vi "AQI SERIAL VISA.vi"() -> ()   [LabVIEW 2023]
uses:
  <vilib>/Instr/_visa.llb/VISA Configure Serial Port (Instr).vi
panel:
  out "MQ7 SENSOR":i32(graph)
  in  "VISA resource name":refnum<visa-resource-name>
  out "read buffer":string
  out "AIR QUALITY SENSOR":dbl(knob) scale=0.0..400.0
  out "GAS METER":dbl(knob) scale=0.0..400.0
  out "CO METER":dbl(slide) scale=0.0..400.0
  out "MQ135 SENSOR":i32(graph)
  out "MQ4 SENSOR":i32(graph)
  in  "STOP":bool
  # "AmanKapil_21001017005"
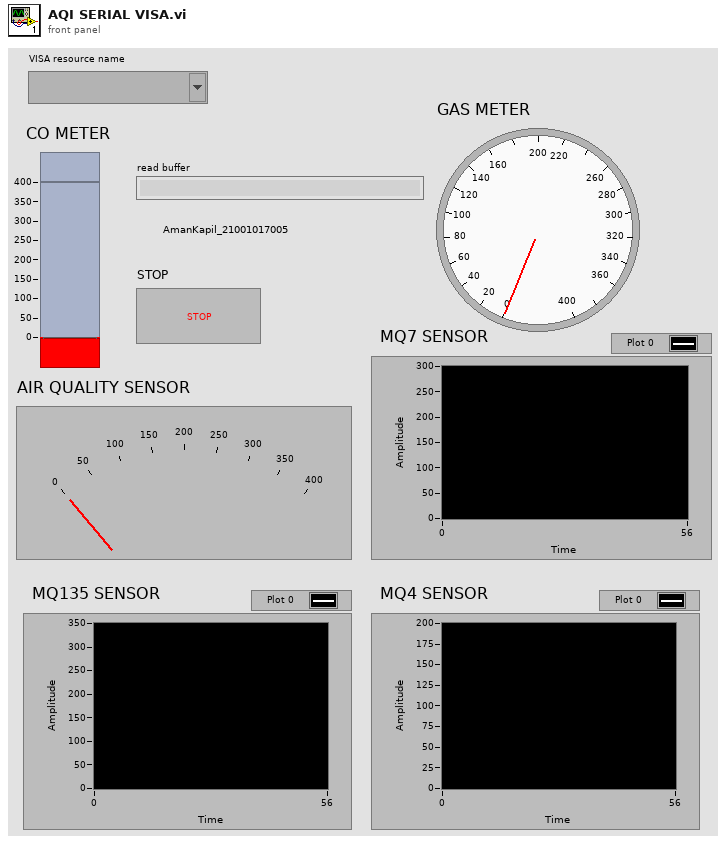
[diagram p1: front panel]
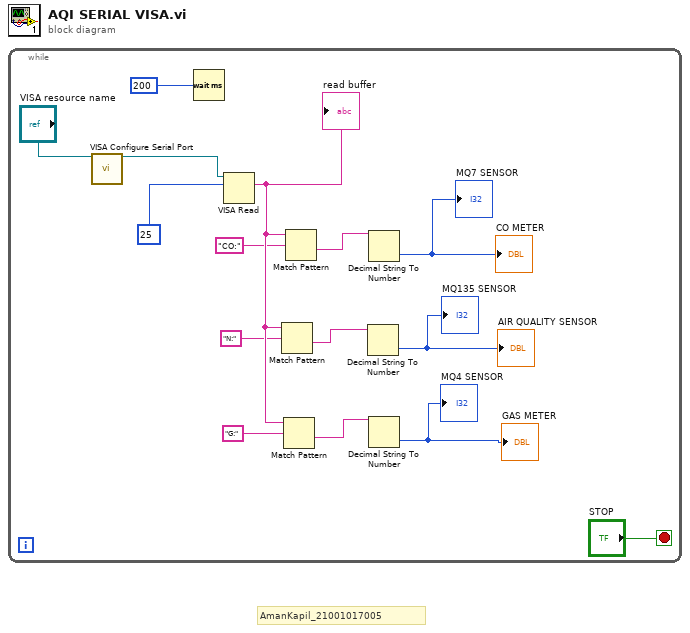
[diagram p0: block diagram]
diagram:
  # "AmanKapil_21001017005"
  n1 = while {
    stop <- "STOP" stop-if-true
    n2 = call-poly "VISA Configure Serial Port"("VISA resource name"="VISA resource name") -> ("VISA resource name out"=w3:refnum<visa-resource-name>)  [unwired: 13 in, 1 out]
    n3 = Wait (ms)(milliseconds to wait=u32 200) -> ()  [unwired: 1 out]
    n4 = VISA Read(VISA resource name=w3, byte count=u32 25) -> (read buffer=w15:string)  [unwired: 1 in, 3 out]
    "read buffer" <- w15
    n5 = Match Pattern(string=w15, regular expression="N:") -> (after substring=w10:string)  [unwired: 1 in, 3 out]
    n6 = Match Pattern(string=w15, regular expression="G:") -> (after substring=w9:string)  [unwired: 1 in, 3 out]
    n7 = Match Pattern(string=w15, regular expression="CO:") -> (after substring=w11:string)  [unwired: 1 in, 3 out]
    n8 = Decimal String To Number(string=w10) -> (number=→"AIR QUALITY SENSOR" →"MQ135 SENSOR":i32)  [unwired: 2 in, 1 out]
    n9 = Decimal String To Number(string=w11) -> (number=→"CO METER" →"MQ7 SENSOR":i32)  [unwired: 2 in, 1 out]
    n10 = Decimal String To Number(string=w9) -> (number=→"GAS METER" →"MQ4 SENSOR":i32)  [unwired: 2 in, 1 out]
  }
